vi "ep_Time Calculation Pt.vi"(0 "multiples of pickup":dbl, 1 "reset delay [s]":dbl, 2 "definite reset? (F)":bool, 5 "time dial":dbl=1.0, 7 "curve parameters":T1={"operate time parameters"={"A [s]"=1.0, "B [s]"=1.0, "alpha"=1.0, "K2 [s]"=1.0, "K1 [s]"=1.0, "K3 [s]"=1.0}, "reset time parameters"={"tr [s]"=1.0, "alpha"=1.0}}, 9 "operate time compensation":cluster{"G/Gs":dbl[], "compensation [s]":dbl[]}, 11 "error in (no error)":errorcluster) -> (4 "compensated time":dbl, 6 "original time":dbl, 15 "error out":errorcluster)   [LabVIEW 2012, in "NI_EP_Protection.lvlib"]
uses:
  <vilib>/addons/Electrical Power/Protection/NI_EP_Protection.lvlib
  <vilib>/addons/Electrical Power/Protection/Inverse Time Delay/subVIs/ep_Curve Parameters.ctl
  <vilib>/addons/Electrical Power/Protection/Inverse Time Delay/subVIs/ep_Operate Time.ctl
  <vilib>/addons/Electrical Power/Protection/Inverse Time Delay/subVIs/ep_Reset Time.ctl
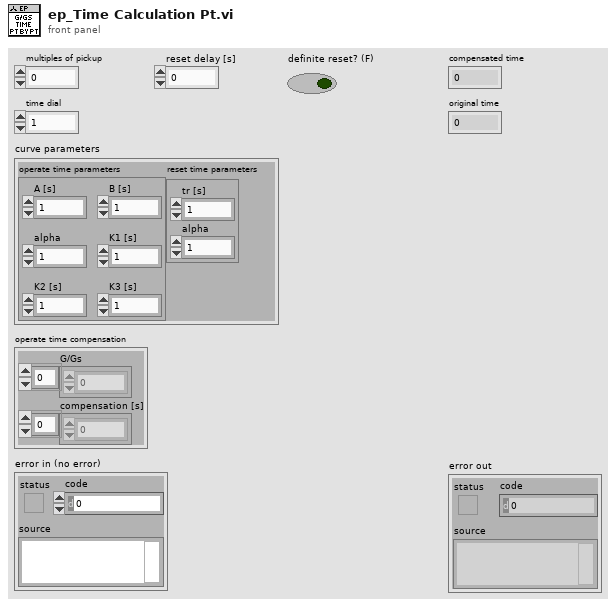
[diagram p1: front panel]
types:
  T1 = typedef "NI_EP_Protection.lvlib/ep_Curve Parameters.ctl" = cluster{"operate time parameters":T2, "reset time parameters":T3}
  T2 = typedef "NI_EP_Protection.lvlib/ep_Operate Time.ctl" = cluster{"A [s]":dbl, "B [s]":dbl, "alpha":dbl, "K2 [s]":dbl, "K1 [s]":dbl, "K3 [s]":dbl}
  T3 = typedef "NI_EP_Protection.lvlib/ep_Reset Time.ctl" = cluster{"tr [s]":dbl, "alpha":dbl}
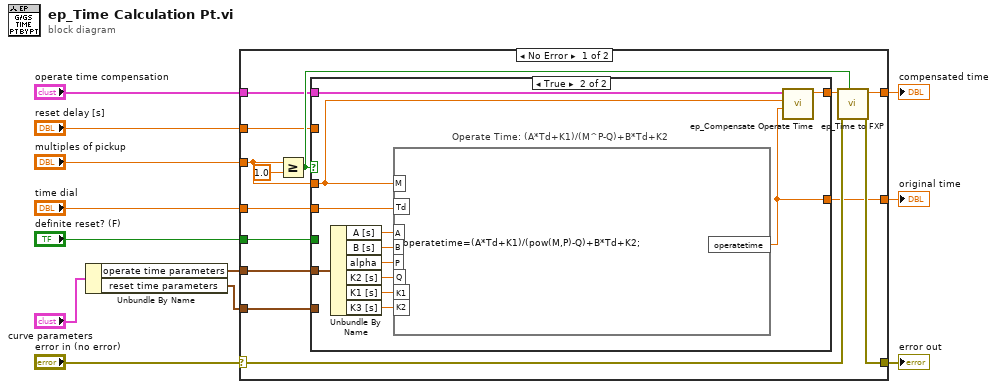
[diagram p0: block diagram]
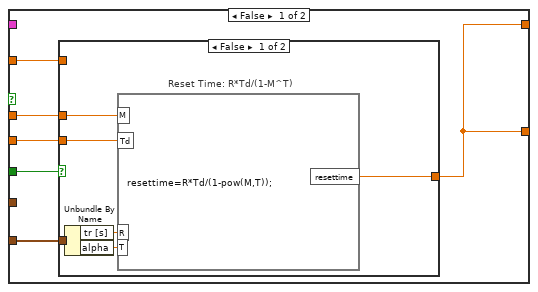
[diagram p2: hidden frame]
diagram:
  n1 = Unbundle By Name("curve parameters") -> ("operate time parameters"=w4:T2, "reset time parameters"=w3:T3)
  n2 = case shown="No Error" "error in (no error)" {
    selector: "error in (no error)" -> [w20 w52]
    tunnel: w4 -> [w26 _]
    tunnel: w3 -> [w25 _]
    tunnel: "time dial" -> [w24 _]
    tunnel: "multiples of pickup" -> [w22 _]
    tunnel: [w19 _] -> w10
    tunnel: [w18 w52] -> w8
    tunnel: "definite reset? (F)" -> [w16 _]
    tunnel: "reset delay [s]" -> [w15 _]
    tunnel: "operate time compensation" -> [w14 _]
    tunnel: [w13 _] -> w1
    frame No Error {
      n3 = Greater Or Equal?(x=w22, y=1.0) -> (x >= y?=w17:bool)
      n4 = case shown="True" w17 {
        tunnel: w26 -> [_ w51]
        tunnel: w25 -> [w32 _]
        tunnel: w22 -> [w31 w43]
        tunnel: w24 -> [w30 w44]
        tunnel: [w27 w41] -> w21
        tunnel: w16 -> [w29 _]
        tunnel: w15 -> [w28 _]
        tunnel: w14 -> [_ w42]
        tunnel: [w27 w40] -> w13
        frame False {
          n5 = case shown="False" w29 {
            tunnel: w32 -> [w38 _]
            tunnel: w31 -> [w35 _]
            tunnel: w30 -> [w34 _]
            tunnel: [w33 w39] -> w27
            tunnel: w28 -> [_ w39]
            frame False {
              # "Reset Time: R*Td/(1-M^T)"
              n6 = Unbundle By Name(w38) -> ("tr [s]"=w37:dbl, "alpha"=w36:dbl)
              n7 = formula code="resettime=R*Td/(1-pow(M,T));"("R"=w37, "T"=w36, "M"=w35, "Td"=w34) -> ("resettime"=w33:dbl)
            }
            frame True {
            }
          }
        }
        frame True {
          # "Operate Time: (A*Td+K1)/(M^P-Q)+B*Td+K2"
          n8 = Unbundle By Name(w51) -> ("A [s]"=w50:dbl, "B [s]"=w49:dbl, "alpha"=w48:dbl, "K2 [s]"=w47:dbl, "K1 [s]"=w46:dbl, "K3 [s]"=w45:dbl)
          n9 = formula code="operatetime=(A*Td+K1)/(pow(M,P)-Q)+B*Td+K2;"("A"=w50, "B"=w49, "P"=w48, "Q"=w47, "K1"=w46, "K2"=w45, "Td"=w44, "M"=w43) -> ("operatetime"=w40:dbl)
          n10 = call <vilib>:"ep_Compensate Operate Time.vi"("operate time"=w40, "multiples of pickup"=w43, "operate time compensation"=w42) -> ("compensated operate time"=w41:dbl)  [unwired: 8 in]
        }
      }
      n11 = call <vilib>:"ep_Time to FXP.vi"("operate?"=w17, "error in (no error)"=w20, "time"=w21) -> ("error out"=w18:errorcluster, "time"=w19:dbl)  [unwired: 7 in]
    }
    frame Error {
    }
  }
  "compensated time" <- w10
  "error out" <- w8
  "original time" <- w1
